vi "mySweepNum.vi"(8 "可以正常测量":bool, 9 "是否有可用DSP":bool, 10 "index group":i32[][](array[numeric]), 11 "注入(1号)端口类型":u8(ring) items=["单相", "三相αβ系", "三相同步系", "三相正负序"]) -> (0 "频点数":i32, 1 "实际使用的注入模式":u8, 2 "M":i32)   [LabVIEW 2024]
doc: "在进入扫频循环之前，计算一些循环相关的参数。\n测试模式：检查能否正常扫频，若不满足，将实际注入模式设成100.\n即，这步补充了“无效配置”时的模式。"
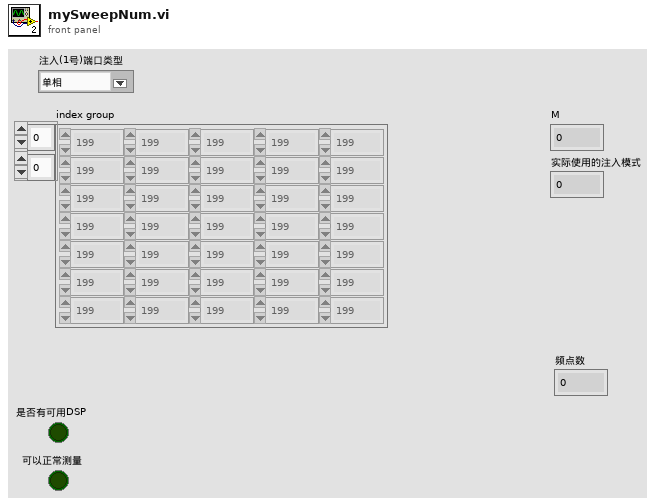
[diagram p1: front panel]
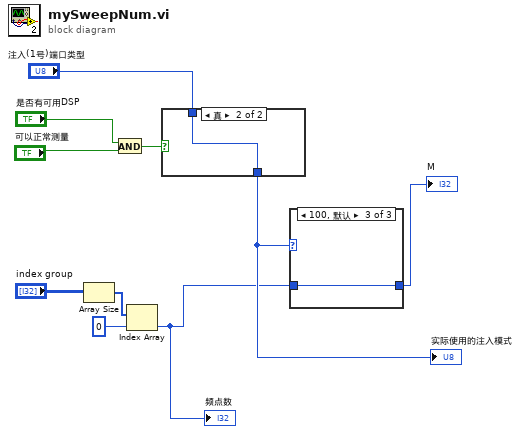
[diagram p0: block diagram]
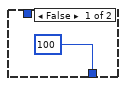
[diagram p2: hidden frame]
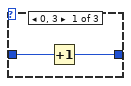
[diagram p3: hidden frame]
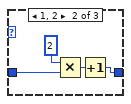
[diagram p4: hidden frame]
diagram:
  n1 = Array Size(array="index group") -> (size(s)=w9:i32[])
  n2 = And(x="是否有可用DSP", y="可以正常测量") -> (x .and. y?=w5:bool)
  n3 = Index Array(array=w9, index=0 ("索引")) -> (element=w2:i32)
  "频点数" <- w2
  n4 = case shown="真" w5 {
    tunnel: "注入(1号)端口类型" -> [_ w12]
    tunnel: [u8 100 w12] -> w3
    frame False {
    }
    frame True {
    }
  }
  "实际使用的注入模式" <- w3
  n5 = case shown="100, 默认" w3 {
    tunnel: [w13 w16 w19] -> w4
    tunnel: w2 -> [w14 w15 w19]
    frame 0, 3 {
      n6 = Increment(x=w14) -> (x+1=w13:i32)
    }
    frame 1, 2 {
      n7 = Multiply(x=2, y=w15) -> (x*y=w18:i32)
      n8 = Increment(x=w18) -> (x+1=w16:i32)
    }
    frame 100, Default {
    }
  }
  "M" <- w4
